vi "isComplete.vi"(8 "error in (no error)":errorcluster, 11 "Drive in":refnum<class "Drive.lvclass">) -> (0 "error out":errorcluster, 2 "Mission Complete?":bool, 3 "Drive out":refnum<class "Drive.lvclass">)   [LabVIEW 2011, in "Drive.lvclass"]
uses:
  Drive.lvclass
  Mission/Mission.lvclass
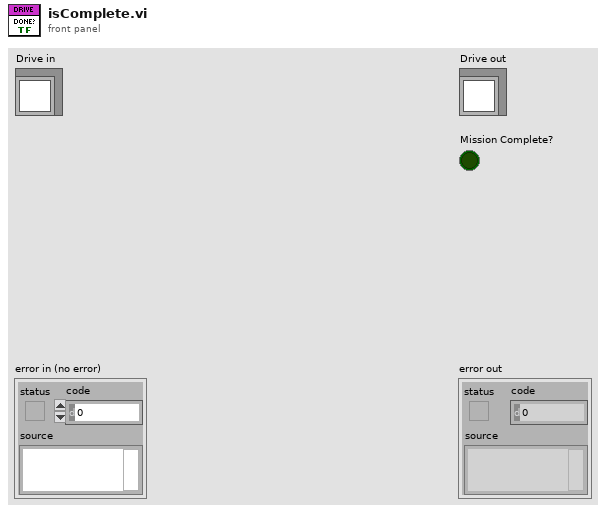
[diagram p1: front panel]
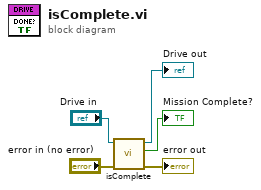
[diagram p0: block diagram]
diagram:
  n1 = call-parent "isComplete.vi"("error in (no error)"="error in (no error)", "Mission in"="Drive in") -> ("error out"=→"error out":errorcluster, "Mission Complete?"=→"Mission Complete?":bool, "Mission out"=→"Drive out":refnum<class "Drive.lvclass">)  [unwired: 7 in]
